vi "sendValue.vi"(8 "error in (no error)":errorcluster, 10 "data":variant, 11 "setRange in":refnum<class "setRange.lvclass">) -> (0 "error out":errorcluster, 2 "function return":i32, 3 "setRange out":refnum<class "setRange.lvclass">)   [LabVIEW 2016, in "SALLV_MtAtElectrometer_Messaging.lvlib" / "setRange.lvclass"]
uses:
  setRange.lvclass
  ts_sallv_MtAtElectrometer/DataTypes/command_setRange.ctl
  ts_sallv_MtAtElectrometer/SALLV_MtAtElectrometer.lvlib
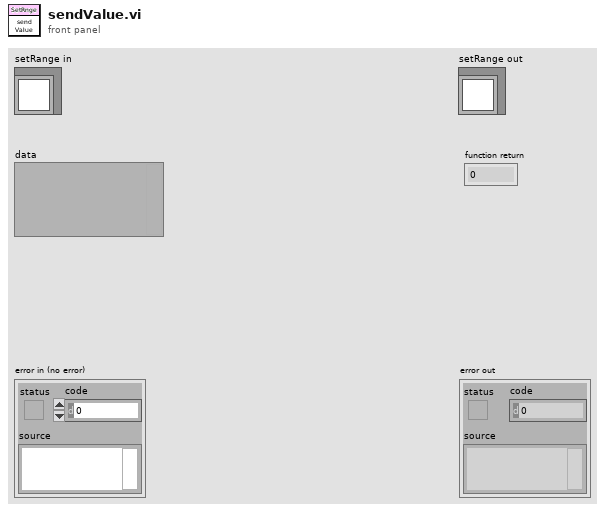
[diagram p1: front panel]
types:
  T1 = typedef "SALLV_MtAtElectrometer.lvlib/command_setRange.ctl" = cluster{"setRange":sgl}
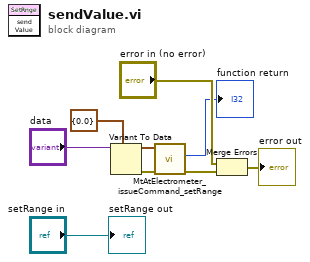
[diagram p0: block diagram]
diagram:
  n1 = Variant To Data(type=T1 {"setRange"=0.0} ("command_setRange_Ctl"), Variant="data") -> (data=w2:T1, error out=w5:errorcluster)  [unwired: 1 in]
  n2 = call "MtAtElectrometer_issueCommand_setRange.vi"("error in (no error)"=w5, "command_setRange_Ctl"=w2) -> ("error out"=w4:errorcluster, "function return"=→"function return":i32)  [unwired: 7 in, 1 out]
  n3 = Merge Errors("error in (no error)", w4) -> (→"error out":errorcluster)
  "setRange out" <- "setRange in"
